vi "OP400ZP_prep bdd NULL.vi"(8 "tabin":string[](array[string])) -> (0 "tabout":string[](array[string]))   [LabVIEW 2020]
uses:
  OP400ZP_selectdata.ctl
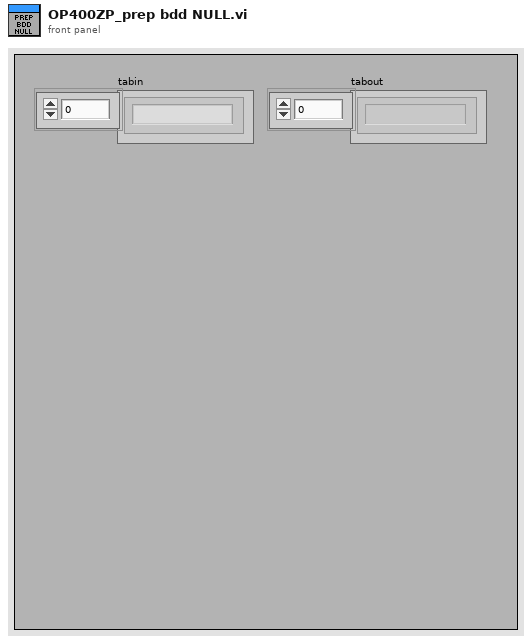
[diagram p1: front panel]
types:
  T1 = typedef "OP400ZP_selectdata.ctl" = u16
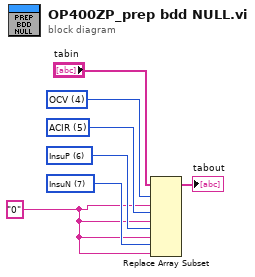
[diagram p0: block diagram]
diagram:
  w1 = "0" ("nouvel élément/sous-tableau")
  w2 = T1 7 items=["IdOp400", "SN", "Type", "DateStart", "OCV", "ACIR", "InsuP", "InsuN", "TC0", "TC1", "DeltaTC", "VC0", "VC1", "DeltaVC", "MCU", "Tfactory", "RefLimite", "IniFileVers", "SoftVers", "ImageVers", "Pass", "Operateur", "TempsTest"] ("Menu déroulant")
  w3 = T1 6 items=["IdOp400", "SN", "Type", "DateStart", "OCV", "ACIR", "InsuP", "InsuN", "TC0", "TC1", "DeltaTC", "VC0", "VC1", "DeltaVC", "MCU", "Tfactory", "RefLimite", "IniFileVers", "SoftVers", "ImageVers", "Pass", "Operateur", "TempsTest"] ("Menu déroulant")
  w4 = T1 5 items=["IdOp400", "SN", "Type", "DateStart", "OCV", "ACIR", "InsuP", "InsuN", "TC0", "TC1", "DeltaTC", "VC0", "VC1", "DeltaVC", "MCU", "Tfactory", "RefLimite", "IniFileVers", "SoftVers", "ImageVers", "Pass", "Operateur", "TempsTest"] ("Menu déroulant")
  w5 = T1 4 items=["IdOp400", "SN", "Type", "DateStart", "OCV", "ACIR", "InsuP", "InsuN", "TC0", "TC1", "DeltaTC", "VC0", "VC1", "DeltaVC", "MCU", "Tfactory", "RefLimite", "IniFileVers", "SoftVers", "ImageVers", "Pass", "Operateur", "TempsTest"] ("Menu déroulant")
  n1 = Replace Array Subset(array="tabin", new element #1=w1, index #1=w5, new element #2=w1, index #2=w4, new element #3=w1, index #3=w3, new element #4=w1, index #4=w2) -> (→"tabout":string[])
